vi "Set Query (array).vi"(8 "error in (no error)":errorcluster, 10 "Query":cluster{"argument":string, "value":string}[](array[cluster]), 11 "URI in":refnum<class "URI.lvclass">) -> (0 "error out":errorcluster, 3 "URI out":refnum<class "URI.lvclass">)   [LabVIEW 2013, in "openURI.lvlib" / "URI.lvclass"]
doc: "The Query variant input must contain attributes of type \"string\".\nAll data contained in the variant will be ignored. All attributes that are not of type \"string\" will be ignored."
uses:
  URI.lvclass
  URI.lvclass/URI.ctl
  components/query/Create Query (array).vi
  checkCached.vi
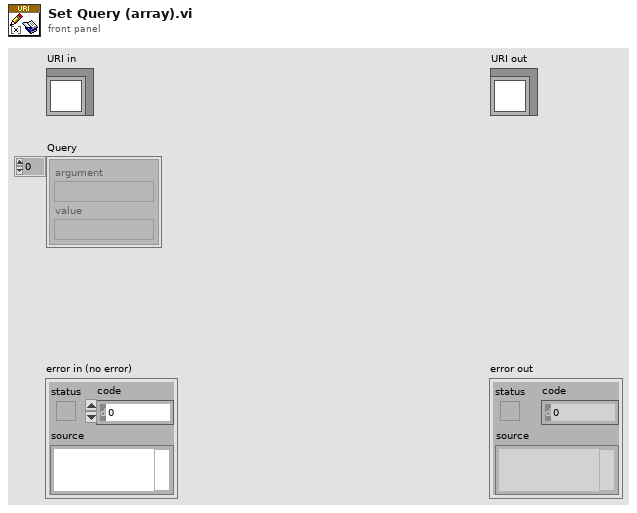
[diagram p1: front panel]
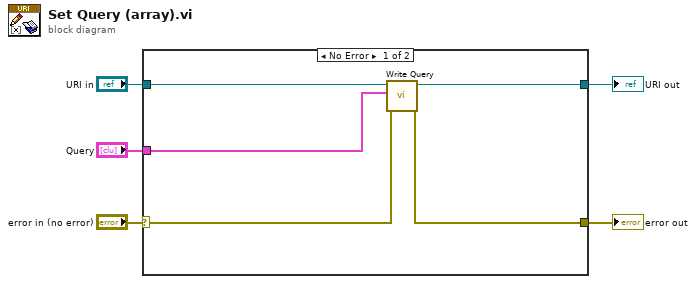
[diagram p0: block diagram]
diagram:
  n1 = case shown="No Error" "error in (no error)" {
    selector: "error in (no error)" -> [w7 w12]
    tunnel: [w8 w12] -> w4
    tunnel: [w9 w11] -> w2
    tunnel: "URI in" -> [w10 w11]
    tunnel: "Query" -> [w6 _]
    frame No Error {
      n2 = call "Write Query.vi"("error in (no error)"=w7, "Query"=w6, "URI in"=w10) -> ("error out"=w8:errorcluster, "URI out"=w9:refnum<class "URI.lvclass">)  [unwired: 7 in]
    }
    frame Error {
    }
  }
  "error out" <- w4
  "URI out" <- w2
